vi "Read Measurement.vi"(8 "error in":errorcluster, 9 "Channel (1: Channel 1)":i32(ring)=1 items=["Channel 1"=1, "Channel 2"=2, "Channel 3"=3, "Channel 4"=4], 10 "Measurement Type (0: Frequency)":i32(ring) items=["Frequency", "Mean", "Period", "Pulse Duty", "Peak to Peak", "Cycle RMS", "Minimum", "Maximum", "Rise Time", "Fall Time", "Positive Width", "Negative Width", "Amplitude", "Cycle Mean", "High", "Low", "Negative Duty", "Positive Overshoot", "Negative Overshoot", "Cursor Mean", "Burst Width", "Positive Pulse Count", "Negative Pulse Count", "Rising Edge Count", "Falling Edge Count", "Area", "Cycle Area", "RMS", "Cursor RMS"], 11 "Tektronic in":refnum<class "Tektronic.lvclass">) -> (0 "error out":errorcluster, 1 "Measurement":dbl, 2 "Units":string, 3 "Tektronic out":refnum<class "Tektronic.lvclass">)   [LabVIEW 2020, in "Controlador.lvlib" / "Tektronic.lvclass"]
uses:
  Tektronic.lvclass
  C:/GitClones/Osciloscope modules/Modulo_Cloneable_DQMH/Libraries/Controlador/Class/Osciloscope/Osciloscope.lvclass
  Osciloscope/Osciloscope.lvclass/Osciloscope.ctl
  Osciloscope/Read COM.vi
  <instrlib>/Tektronix TDS 200 1000 2000 Series/Tektronix TDS 200 1000 2000 Series.lvlib
  Osciloscope/Osciloscope.lvclass
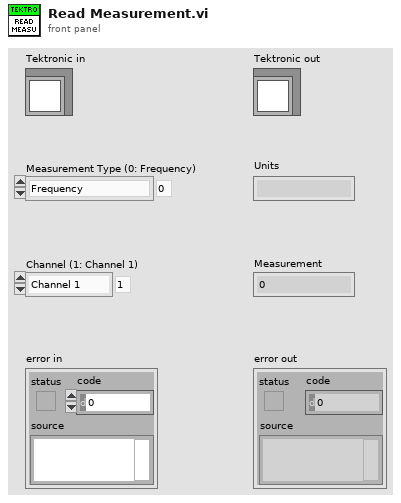
[diagram p1: front panel]
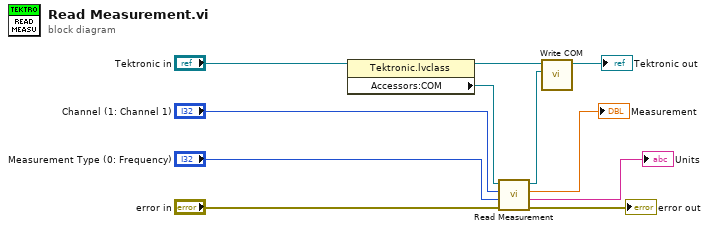
[diagram p0: block diagram]
diagram:
  n1 = property class="Tektronic.lvclass"(reference="Tektronic in") -> (reference out=w3:refnum<class "Tektronic.lvclass">, "Accessors:COM"=w4:refnum<visa-resource-name>)  [unwired: 1 in, 1 out]
  n2 = call <instrlib>:"Read Measurement.vi"("error in (no error)"="error in", "Measurement Type (0: Frequency)"="Measurement Type (0: Frequency)", "Channel (1: Channel 1)"="Channel (1: Channel 1)", "VISA resource name"=w4) -> ("error out"=→"error out":errorcluster, "Units"=→"Units":string, "Measurement"=→"Measurement":dbl, "VISA resource name out"=w2:refnum<visa-resource-name>)  [unwired: 4 in]
  n3 = call "Write COM.vi"("COM"=w2, "Osciloscope in"=w3) -> ("Osciloscope out"=→"Tektronic out":refnum<class "Tektronic.lvclass">)  [unwired: 8 in, 1 out]
